vi "Draw Tip.vi"(8 "error in (no error)":errorcluster, 10 "Adjusted Coordinate":cluster{dbl, dbl}, 11 "Refnum in":T1) -> (0 "error out":errorcluster, 3 "Refnum out":T1)   [LabVIEW 2016]
doc: "This VI draws the tip's position on an image."
uses:
  <vilib>/vision/Image Controls.llb/IMAQ Image.ctl
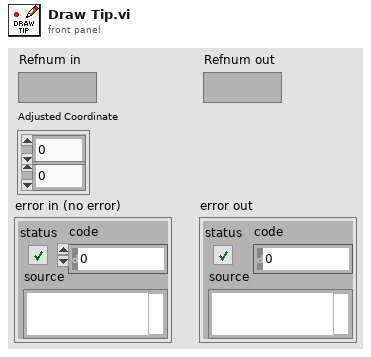
[diagram p1: front panel]
types:
  T1 = typedef "IMAQ Image.ctl" = refnum<image>
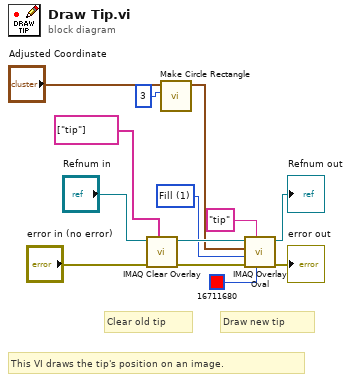
[diagram p0: block diagram]
diagram:
  w2 = u32 1 items=["Frame", "Fill"] ("Drawing Mode (Frame)")
  # "This VI draws the tip's position on an image."
  # "Draw new tip"
  # "Clear old tip"
  n1 = call "IMAQ Clear Overlay"("Groups"=string[] ["tip"], "error in (no error)"="error in (no error)", "Image"="Refnum in") -> ("error out"=w9:errorcluster, "Image Out"=w8:T1)  [unwired: 7 in]
  n2 = call "Make Circle Rectangle.vi"("Size"=3, "Coordinate"="Adjusted Coordinate") -> ("Rectangle"=w4:cluster{dbl, dbl, dbl, dbl})  [unwired: 9 in]
  n3 = call "IMAQ Overlay Oval"("Color"=u32 16711680, "Group"="tip", "error in (no error)"=w9, "Drawing Mode (Frame)"=w2, "Bounding Rectangle"=w4, "Image"=w8) -> ("error out"=→"error out":errorcluster, "Image Out"=→"Refnum out":T1)  [unwired: 4 in]
